vi "ConvertCameraCoords.vi"(11 "ion coords":T1={"Top :"=103.0, "Bottom :"=100.0, "Left :"=100.0, "Right :"=103.0}) -> (3 "subimage cluster":T2)   [LabVIEW 2019]
uses:
  CameraCoordsControl.ctl
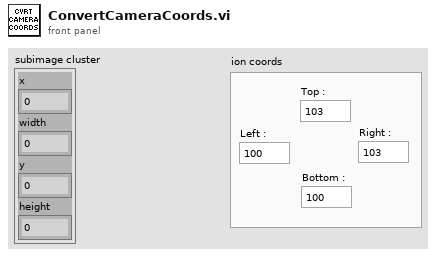
[diagram p1: front panel]
types:
  T1 = typedef "CameraCoordsControl.ctl" = cluster{"Top :":dbl, "Bottom :":dbl, "Left :":dbl, "Right :":dbl}
  T2 = cluster{"x":i32, "width":i32, "y":i32, "height":i32}
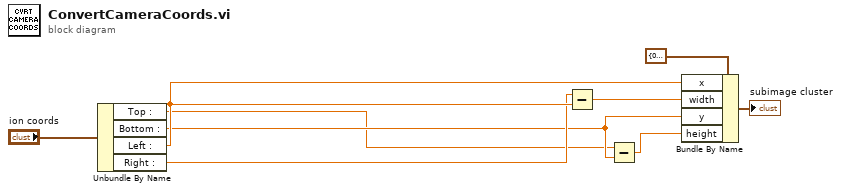
[diagram p0: block diagram]
diagram:
  n1 = Unbundle By Name("ion coords") -> ("Top :"=w1:dbl, "Bottom :"=w2:dbl, "Left :"=w4:dbl, "Right :"=w3:dbl)
  n2 = Subtract(x=w3, y=w4) -> (x-y=w6:dbl)
  n3 = Subtract(x=w1, y=w2) -> (x-y=w5:dbl)
  n4 = Bundle By Name(cluster=T2 {"x"=0, "width"=0, "y"=0, "height"=0} ("subimage cluster 2"), "x"=w4, "width"=w6, "y"=w2, "height"=w5) -> (→"subimage cluster":T2)
